vi "WRITE.vi"(8 "error in (no error)":errorcluster, 10 "Monedas 3":T1(array[cluster])) -> (0 "error out":errorcluster)   [LabVIEW 2020, in "Monedas.lvlib"]
uses:
  Monedas.lvlib
  <vilib>/Utility/xml.llb/Write to XML File(string).vi
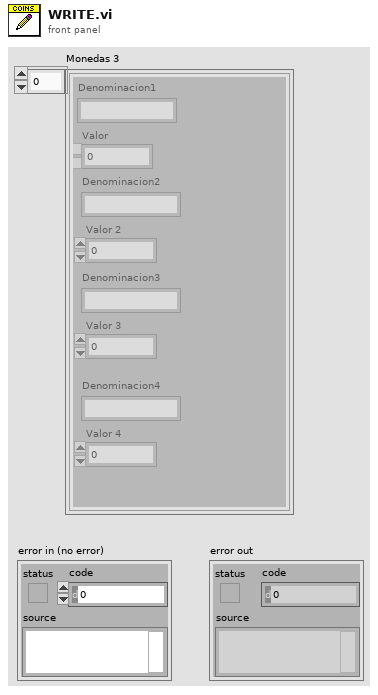
[diagram p1: front panel]
types:
  T1 = cluster{"Denominacion1":string, "Valor":dbl, "Denominacion2":string, "Valor 2":dbl, "Denominacion3":string, "Valor 3":dbl, "Denominacion4":string, "Valor 4":dbl}[]
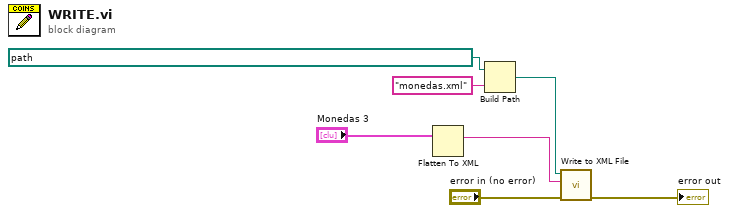
[diagram p0: block diagram]
diagram:
  n1 = Flatten To XML(6:"Monedas 3") -> (2:w5:string)
  n2 = Build Path(base path=path "C:/Users/Ymata/Desktop/séptimo/labview 7mo/Proyecto máuina/Proyecto-maquina", name or relative path="monedas.xml") -> (appended path=w2:path)
  n3 = call-poly <vilib>:"Write to XML File.vi"("error in (no error)"="error in (no error)", "XML Input"=w5, "XML File Path"=w2) -> ("error out"=→"error out":errorcluster)  [unwired: 6 in, 2 out]
